vi "通讯全局变量断电保存.vi"() -> ()   [LabVIEW 2016, in "环境动力单元.lvlib"]
panel:
  in  "排气扇参数":T1={"功能开关"=enum."关闭", "排气扇开启温度"=60.0, "排气扇关闭温度"=60.0}
  in  "冰箱参数":T2={"功能开关"=enum."关闭", "开启时间"=2, "关闭时间"=2} {"关闭时间" items=["00H", "01H", "02H", "03H", "04H", "05H", "06H", "07H", "08H", "09H", "10H", "11H", "12H", "13H", "14H", "15H", "16H", "17H", "18H", "19H", "20H", "21H", "22H", "23H", "关闭"]; "开启时间" items=["00H", "01H", "02H", "03H", "04H", "05H", "06H", "07H", "08H", "09H", "10H", "11H", "12H", "13H", "14H", "15H", "16H", "17H", "18H", "19H", "20H", "21H", "22H", "23H", "关闭"]}
  in  "采配水参数":T3={"排空时间"=60.0, "润洗时间"=60.0, "进样超时时间"=300.0, "沉淀时间"=1800.0}
  in  "运行周期":T4
  in  "MPPT-24 启用":bool
  in  "MPPT-24 Serial":refnum<visa-resource-name>
  in  "MPPT-12 启用":bool
  in  "MPPT-12 Serial":refnum<visa-resource-name>
  in  "ZLAN 启用":bool=TRUE
  in  "ZLAN IP":string="192.168.1.200"
  in  "报警参数配置":T5={"低压报警阈值 V"=22.0, "低压报警解除阈值 V"=25.0, "高温报警阈值 ℃"=50.0, "高温报警解除阈值 ℃"=40.0, "湿度报警阈值 %"=95.0, "湿度报警解除阈值 %"=90.0}
  out "工程量转换":T6={"原始值最小值"=0.0, "原始值最大值"=65535.0, "转换值最小值"=0.0, "转换值最大值"=10.0, "原始值最小值 2"=0.0, "原始值最大值 2"=65535.0, "转换值最小值 2"=0.0, "转换值最大值 2"=10.0, "原始值最小值 3"=0.0, "原始值最大值 3"=65535.0, "转换值最小值 3"=0.0, "转换值最大值 3"=10.0, "原始值最小值 4"=0.0, "原始值最大值 4"=65535.0, "转换值最小值 4"=0.0, "转换值最大值 4"=10.0, "原始值最小值 5"=0.0, "原始值最大值 5"=65535.0, "转换值最小值 5"=0.0, "转换值最大值 5"=10.0, "原始值最小值 6"=0.0, "原始值最大值 6"=65535.0, "转换值最小值 6"=0.0, "转换值最大值 6"=10.0, "原始值最小值 7"=0.0, "原始值最大值 7"=65535.0, "转换值最小值 7"=0.0, "转换值最大值 7"=10.0, "原始值最小值 8"=0.0, "原始值最大值 8"=65535.0, "转换值最小值 8"=0.0, "转换值最大值 8"=10.0} {"转换值最大值 8" format="%#.2f"; "转换值最小值 8" format="%#.2f"; "原始值最大值 8" format="%#.2f"; "原始值最小值 8" format="%#.2f"; "转换值最大值 7" format="%#.2f"; "转换值最小值 7" format="%#.2f"; "原始值最大值 7" format="%#.2f"; "原始值最小值 7" format="%#.2f"; "转换值最大值 6" format="%#.2f"; "转换值最小值 6" format="%#.2f"; "原始值最大值 6" format="%#.2f"; "原始值最小值 6" format="%#.2f"; "转换值最大值 5" format="%#.2f"; "转换值最小值 5" format="%#.2f"; "原始值最大值 5" format="%#.2f"; "原始值最小值 5" format="%#.2f"; "转换值最大值 4" format="%#.2f"; "转换值最小值 4" format="%#.2f"; "原始值最大值 4" format="%#.2f"; "原始值最小值 4" format="%#.2f"; "转换值最大值 3" format="%#.2f"; "转换值最小值 3" format="%#.2f"; "原始值最大值 3" format="%#.2f"; "原始值最小值 3" format="%#.2f"; "转换值最大值 2" format="%#.2f"; "转换值最小值 2" format="%#.2f"; "原始值最大值 2" format="%#.2f"; "原始值最小值 2" format="%#.2f"; "转换值最大值" format="%#.2f"; "转换值最小值" format="%#.2f"; "原始值最大值" format="%#.2f"; "原始值最小值" format="%#.2f"}
  # "运行模式："
  # "原始低值"
  # "原始高值"
  # "转换低值"
  # "转换高值"
  # "AD7:"
  # "AD6:"
  # "AD5:"
  # "AD4:"
  # "AD3:"
  # "AD2:"
  # "AD1:"
  # "AD0:"
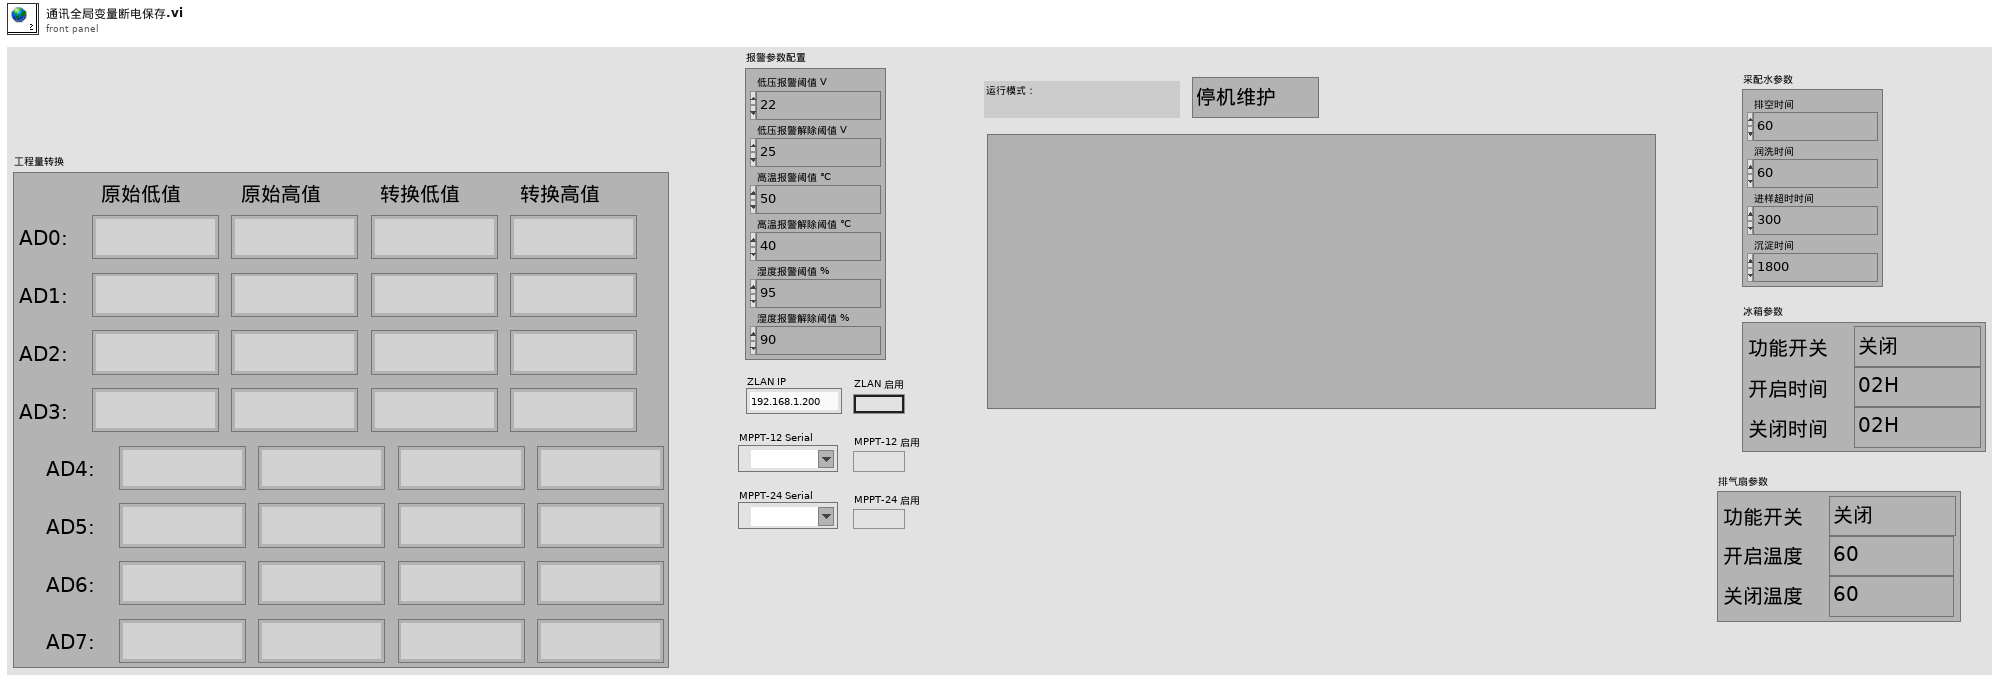
[diagram p1: front panel]
types:
  T1 = cluster{"功能开关":enum16{"关闭", "开启"}, "排气扇开启温度":dbl, "排气扇关闭温度":dbl}
  T2 = cluster{"功能开关":enum16{"关闭", "开启"}, "开启时间":u16, "关闭时间":u16}
  T3 = cluster{"排空时间":dbl, "润洗时间":dbl, "进样超时时间":dbl, "沉淀时间":dbl}
  T4 = cluster{"运行模式":enum16{"停机维护", "正常运行"}, "24H周期设置":bool[]}
  T5 = cluster{"低压报警阈值 V":dbl, "低压报警解除阈值 V":dbl, "高温报警阈值 ℃":dbl, "高温报警解除阈值 ℃":dbl, "湿度报警阈值 %":dbl, "湿度报警解除阈值 %":dbl}
  T6 = cluster{"原始值最小值":dbl, "原始值最大值":dbl, "转换值最小值":dbl, "转换值最大值":dbl, "原始值最小值 2":dbl, "原始值最大值 2":dbl, "转换值最小值 2":dbl, "转换值最大值 2":dbl, "原始值最小值 3":dbl, "原始值最大值 3":dbl, "转换值最小值 3":dbl, "转换值最大值 3":dbl, "原始值最小值 4":dbl, "原始值最大值 4":dbl, "转换值最小值 4":dbl, "转换值最大值 4":dbl, "原始值最小值 5":dbl, "原始值最大值 5":dbl, "转换值最小值 5":dbl, "转换值最大值 5":dbl, "原始值最小值 6":dbl, "原始值最大值 6":dbl, "转换值最小值 6":dbl, "转换值最大值 6":dbl, "原始值最小值 7":dbl, "原始值最大值 7":dbl, "转换值最小值 7":dbl, "转换值最大值 7":dbl, "原始值最小值 8":dbl, "原始值最大值 8":dbl, "转换值最小值 8":dbl, "转换值最大值 8":dbl}
diagram:
